vi "ReadConfig.vi"(8 "error in (no error)":errorcluster, 11 "QuickNote in":refnum<class "QuickNote.lvclass">) -> (0 "error out":errorcluster, 3 "QuickNote out":refnum<class "QuickNote.lvclass">)   [LabVIEW 2020, in "QuickNote.lvlib" / "QuickNote.lvclass"]
uses:
  QuickNote.lvclass
  QuickNote.lvclass/QuickNote.ctl
  Hardware Abstraction Layer/Component/GenericActor/GenericActor/GenericController.lvclass
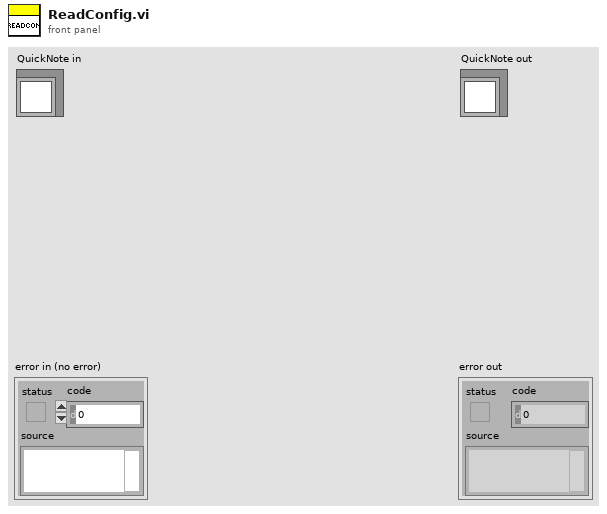
[diagram p1: front panel]
types:
  T1 = typedef "NI_LVConfig.lvlib/Config Data RefNum.ctl" = refnum<k1>
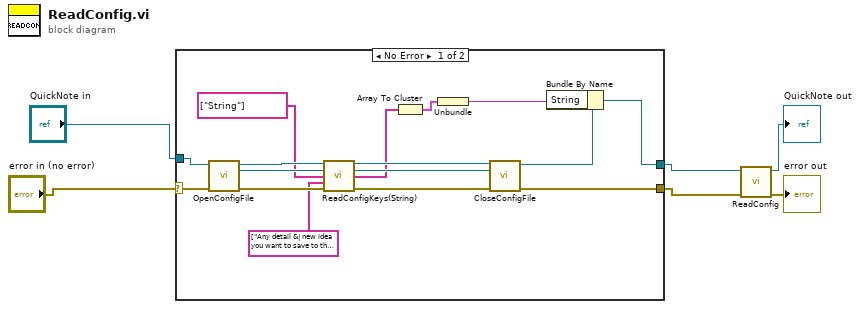
[diagram p0: block diagram]
diagram:
  n1 = case shown="No Error" "error in (no error)" {
    selector: "error in (no error)" -> [w22 w23]
    tunnel: [w14 w23] -> w1
    tunnel: [w17 w24] -> w2
    tunnel: "QuickNote in" -> [w21 w24]
    frame No Error {
      n2 = call-dynamic "OpenConfigFile.vi"("error in (no error)"=w22, "GRMActor in"=w21) -> ("error out"=w20:errorcluster, "refnum"=w15:T1, "GRMActor out"=w18:refnum<class "QuickNote.lvclass">)  [unwired: 7 in]
      n3 = call-dynamic "ReadConfigKeys(String).vi"("GRMActor in"=w18, "Config Refnum"=w15, "Keys"=string[] ["String"] ("Values"), "Values"=string[] ["Any detail &| new idea you want to save to the image folder?"], "error in (no error)"=w20) -> ("GRMActor out"=w13:refnum<class "QuickNote.lvclass">, "Config Refnum dup"=w10:T1, "Values"=w9:string[], "error out"=w19:errorcluster)  [unwired: 7 in]
      n4 = Array To Cluster(array=w9) -> (cluster=w16:cluster{"Values[0]":string})
      n5 = Unbundle(w16) -> ("Values[0]"=w11:string)
      n6 = call-dynamic "CloseConfigFile.vi"("error in (no error)"=w19, "refnum"=w10, "GRMActor in"=w13) -> ("error out"=w14:errorcluster, "GRMActor out"=w12:refnum<class "QuickNote.lvclass">)  [unwired: 7 in]
      n7 = Bundle By Name(cluster=w12, "String"=w11) -> (w17:refnum<class "QuickNote.lvclass">)
    }
    frame Error {
    }
  }
  n8 = call-parent "ReadConfig.vi"("error in (no error)"=w1, "GRMActor in"=w2) -> ("error out"=→"error out":errorcluster, "GRMActor out"=→"QuickNote out":refnum<class "QuickNote.lvclass">)  [unwired: 8 in]
